vi "Packet_generator.vi"(9 "Message Bits":i32, 10 "Samples pr burst":i32, 11 "user  bitstream":i8[](array[numeric])=[1]) -> (3 "Array":i8[][](array[numeric]))   [LabVIEW 2014]
uses:
  <vilib>/addons/Modulation/Digital/General/MT Generate Bits (Galois, PN Order).vi
  <vilib>/addons/Modulation/Digital/Support/Common/Validators/mod_Generate Bits Validate.vi
  <vilib>/addons/Modulation/Analog/support/mod_Set Error Source.vi
  <vilib>/addons/Modulation/Digital/General/subVIs/mod_Generate Bits PN Sequence.vi
  <vilib>/addons/Modulation/niDMT.lvlib
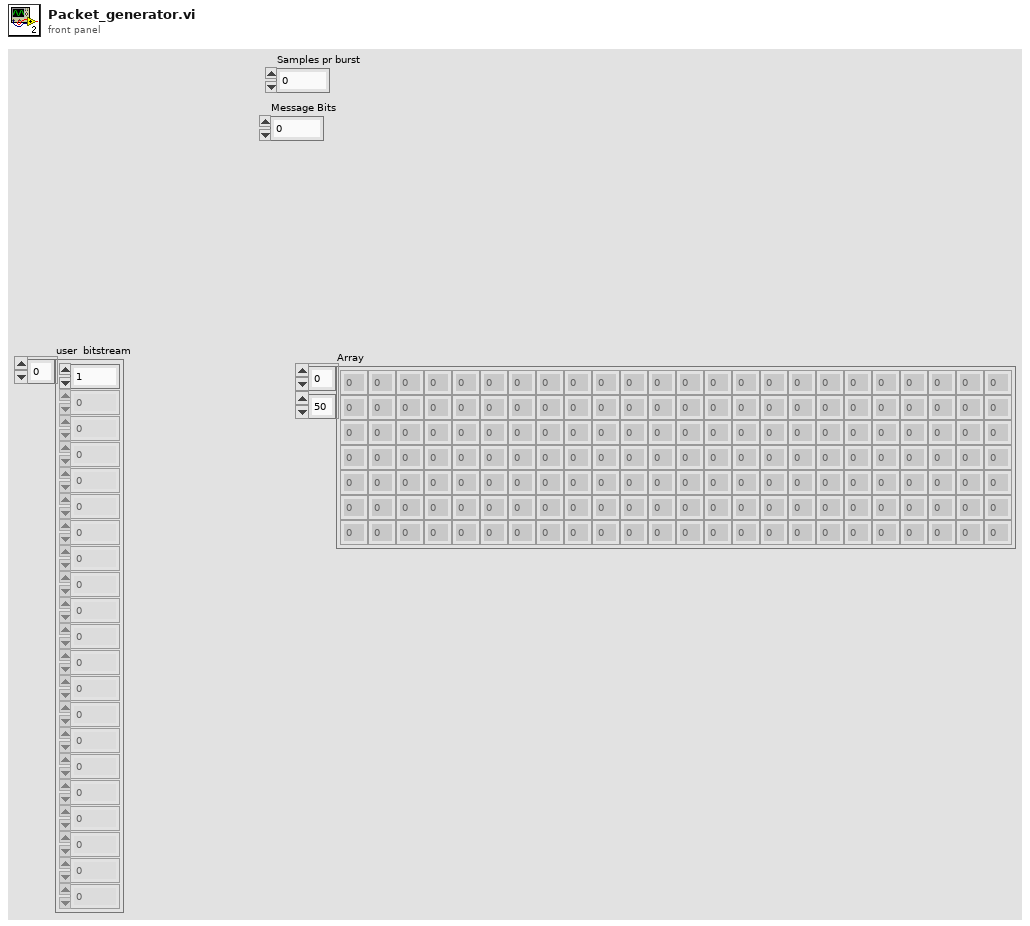
[diagram p1: front panel]
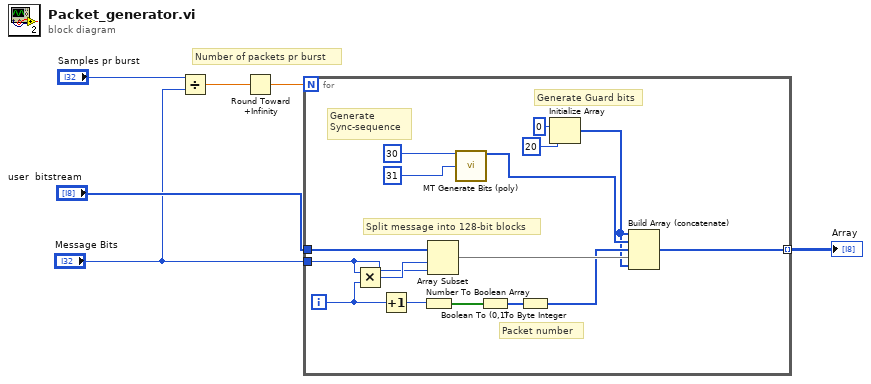
[diagram p0: block diagram]
diagram:
  # "Number of packets pr burst"
  n1 = Divide(x="Samples pr burst", y="Message Bits") -> (x/y=w2:dbl)
  n2 = Round Toward +Infinity(x=w2) -> (ceil(x): smallest int >= x=w1:dbl)
  n3 = for {
    N: w1 -> [_]
    tunnel: "Message Bits" -> [w15]
    tunnel: "user  bitstream" -> [w16]
    tunnel: [w22] -> w5 mode=indexing
    i -> [w7]
    # "Split message into 128-bit blocks"
    # "Packet number"
    # "Generate Guard bits"
    # "Generate\nSync-sequence"
    n4 = Multiply(x=w15, y=w7) -> (x*y=w17:i32)
    n5 = Increment(x=w7) -> (x+1=w18:i32)
    n6 = Number To Boolean Array(number=w18) -> (Boolean array=w19:bool[])
    n7 = Array Subset(array=w16, index=w17, length=w15) -> (w14:i8[])
    n8 = call-poly <vilib>:"MT Generate Bits (poly).vi"("total bits (128)"=30, "PN sequence order (9)"=31) -> ("output bit stream"=w12:i8[])  [unwired: 11 in, 2 out]
    n9 = Boolean To (0,1)(Boolean=w19) -> (0, 1=w20:i16[])
    n10 = To Byte Integer(number=w20) -> (8bit integer=w13:i8[])
    n11 = Initialize Array(0 ("Numeric"), 20 ("dimension size")) -> (w9:i32[])
    n12 = Build Array (concatenate)(w9, w12, w13, w14, w9) -> (w22:i32[])
  }
  "Array" <- w5
